vi "image_reader.vi"(11 "input image 2":path) -> (3 "Image 2":T1(plugin-control))   [LabVIEW 2021]
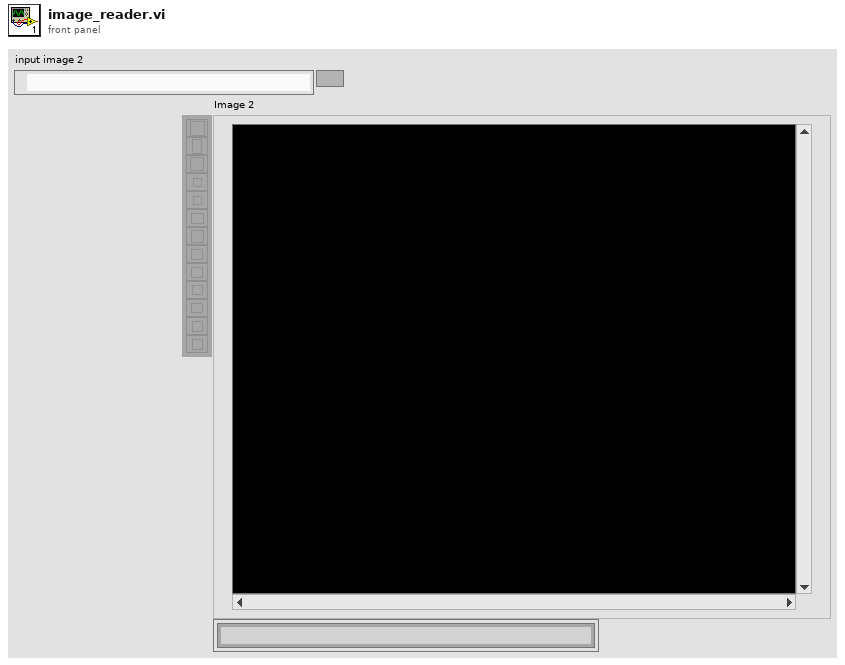
[diagram p1: front panel]
types:
  T1 = typedef "IMAQ Image.ctl" = refnum<image>
  T2 = typedef "Image Type" = u32
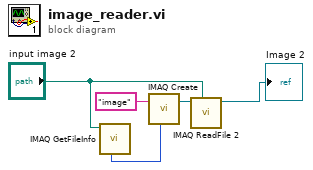
[diagram p0: block diagram]
diagram:
  n1 = call "IMAQ GetFileInfo"("File Path"="input image 2") -> ("Image Type"=w3:T2)  [unwired: 4 in, 6 out]
  n2 = call "IMAQ Create"("Image Name"="image", "Image Type"=w3) -> ("New Image"=w2:T1)  [unwired: 3 in, 1 out]
  n3 = call "IMAQ ReadFile 2"("File Path"="input image 2", "Image"=w2) -> ("Image Out"=→"Image 2":T1)  [unwired: 5 in, 4 out]
